vi "20T_Queue_Commands.vi"(1 "20T Control (in)":T1={"Clamp"=FALSE, "Switch Heater"=FALSE, "Go to Zero"=FALSE, "Go to Set"=FALSE, "Go to Hold"=FALSE, "Setpoint (T)"=3.4572, "Rate (T/min)"=0.0, "Set Rate"=FALSE} {"Rate (T/min)" format="%6_5f"; "Setpoint (T)" format="%#4_5f"}, 3 "20T Queue":refnum<queue>) -> (0 "20T Control (out)":T1={"Clamp"=FALSE, "Switch Heater"=FALSE, "Go to Zero"=FALSE, "Go to Set"=FALSE, "Go to Hold"=FALSE, "Setpoint (T)"=3.4572, "Rate (T/min)"=0.0, "Set Rate"=FALSE} {"Rate (T/min)" format="%6_5f"; "Setpoint (T)" format="%#4_5f"})   [LabVIEW 2019]
uses:
  Gustav/20T_Control.ctl
panel:
  # "20 T"
  # "20 T"
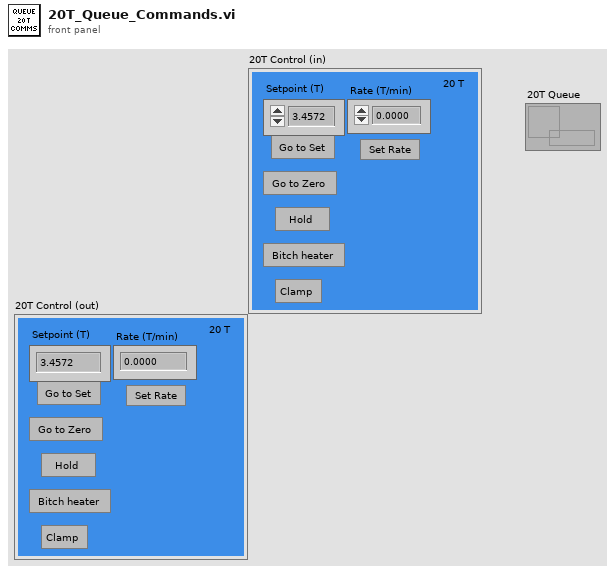
[diagram p1: front panel]
types:
  T1 = typedef "20T_Control.ctl" = cluster{"Clamp":bool, "Switch Heater":bool, "Go to Zero":bool, "Go to Set":bool, "Go to Hold":bool, "Setpoint (T)":dbl, "Rate (T/min)":dbl, "Set Rate":bool}
  T2 = cluster{"Clamp":bool, "Switch Heater":bool, "Go to Zero":bool, "Go to Set":bool, "Go to Hold":bool, "Setpoint (T)":bool, "Rate (T/min)":bool, "Set Rate":bool}
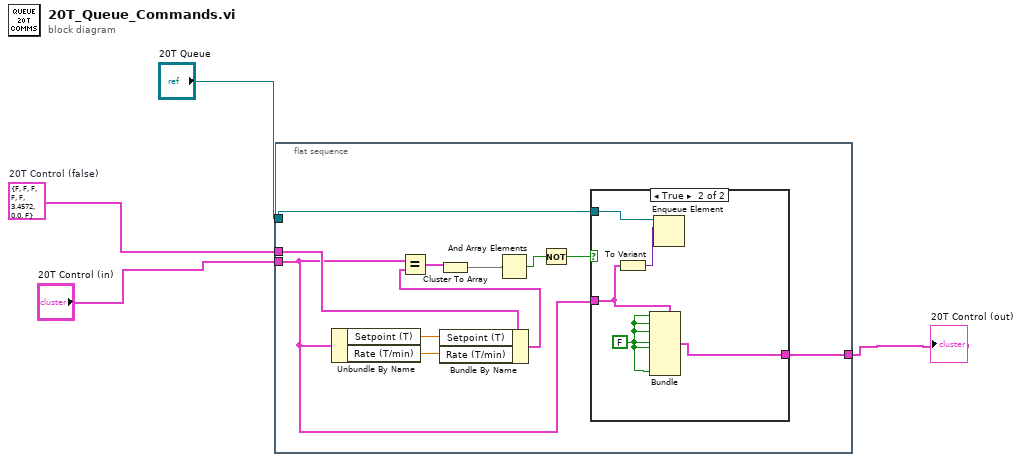
[diagram p0: block diagram]
diagram:
  w1 = T1 {"Clamp"=FALSE, "Switch Heater"=FALSE, "Go to Zero"=FALSE, "Go to Set"=FALSE, "Go to Hold"=FALSE, "Setpoint (T)"=3.4572, "Rate (T/min)"=0.0, "Set Rate"=FALSE}  # 20T Control (false)
  n1 = flat-sequence {
    tunnel: "20T Queue" -> [w15]
    tunnel: "20T Control (in)" -> [w5]
    tunnel: w1 -> [w9]
    tunnel: [w10] -> w2
    frame #0 {
      n2 = Unbundle By Name(w5) -> ("Setpoint (T)"=w8:dbl, "Rate (T/min)"=w7:dbl)
      n3 = Bundle By Name(cluster=w9, "Setpoint (T)"=w8, "Rate (T/min)"=w7) -> (w6:T1)
      n4 = Equal?(x=w5, y=w6) -> (x = y?=w11:T2)
      n5 = Cluster To Array(cluster=w11) -> (array=w14:bool[])
      n6 = And Array Elements(Boolean array=w14) -> (logical AND=w13:bool)
      n7 = Not(x=w13) -> (.not. x?=w12:bool)
      n8 = case shown="True" w12 {
        tunnel: w15 -> [_ w21]
        tunnel: w5 -> [w16 w19]
        tunnel: [w16 w18] -> w10
        frame False {
        }
        frame True {
          w17 = FALSE
          n9 = To Variant(anything=w19) -> (Variant=w20:variant)
          n10 = Bundle(cluster=w19, "Clamp"=w17, "Switch Heater"=w17, "Go to Zero"=w17, "Go to Set"=w17, "Go to Hold"=w17, "Set Rate"=w17) -> (w18:T1)  [unwired: 2 in]
          n11 = Enqueue Element(queue=w21, element=w20) -> ()  [unwired: 2 in, 3 out]
        }
      }
    }
  }
  "20T Control (out)" <- w2
